vi "SR Scan.vi"() -> ()   [LabVIEW 2012]
uses:
  user.lib/SpectralRadar.llb/Scan Pattern.lvclass
  user.lib/SpectralRadar.llb/Probe.lvclass
  user.lib/SpectralRadar.llb/Coloring.lvclass
  user.lib/SpectralRadar.llb/Colorscheme Selection.ctl
  user.lib/SpectralRadar.llb/ImageField.lvclass
  <vilib>/Utility/error.llb/DialogType.ctl
  user.lib/SpectralRadar.llb/Coloring Byteorder.ctl
  user.lib/SpectralRadar.llb/Probe Parameter Int Selection.ctl
  user.lib/SpectralRadar.llb/Processing Parameter Int Selection.ctl
  user.lib/SpectralRadar.llb/Normal Direction Selection.ctl
  user.lib/SpectralRadar.llb/Colored Data Export Format Selection.ctl
  user.lib/SpectralRadar.llb/Data Export Format Selection.ctl
  user.lib/SpectralRadar.llb/Data Analyzation Selection.ctl
  user.lib/SpectralRadar.llb/display Data 2D.vi
  user.lib/SpectralRadar.llb/display Data 1D in XY-Graph.vi
  user.lib/SpectralRadar.llb/set Scan Output.vi
  user.lib/SpectralRadar.llb/Colored Data.lvclass
  user.lib/SpectralRadar.llb/LabVIEW Helper.lvlib
  user.lib/SpectralRadar.llb/OCT Device.lvclass
  user.lib/SpectralRadar.llb/Processing.lvclass
  user.lib/SpectralRadar.llb/FullRange.lvclass
  user.lib/SpectralRadar.llb/Settings.lvclass
  user.lib/SpectralRadar.llb/FileSelection.lvlib
  user.lib/SpectralRadar.llb/Raw Data.lvclass
  user.lib/SpectralRadar.llb/Data.lvclass
  user.lib/SpectralRadar.llb/Buffer.lvclass
  user.lib/SpectralRadar.llb/Post Processing.lvlib
  user.lib/SpectralRadar.llb/Raw Data Export Format Selection.ctl
panel:
  in  "Average A-scan":bool
  in  "Boolean 2":bool
  in  "Filter Options":bool
  in  "Filter":bool
  in  "B-Scan \nAveraging":i32=1 min=1 max=20 step=1
  in  "BScan angle \n[deg]":dbl(knob) scale=0.0..180.0 scale format="%#.6g"
  in  "BScan\nY offset [mm]":dbl min=-5.0 max=5.0 format="%_4f"
  in  "BScan\nX offset [mm]":dbl min=-5.0 max=5.0 format="%_4f"
  out "ImageField":refnum<class "ImageField.lvclass">
  in  "Auto Range Button":bool
  in  "Image field correction":bool
  out "Save All Progress":i32(slide) min=0 max=35 scale=0.0..11.0
  in  "Palette":T1
  in  "Light":dbl(slide)=51.27999885380268 caption="Sharpness" min=0.0 max=100.0 step=0.009999999776482582 scale=0.0..100.0
  out "Coloring":refnum<class "Coloring.lvclass">
  out "GalvoControl":refnum<class "Probe.lvclass">
  out "Scan Pattern":refnum<class "Scan Pattern.lvclass">
  out "AutoSafe":bool
  in  "Stability":dbl(slide) caption="SNR" min=0.0 max=1.0 step=1.0
  in  "Averaging*Binning":i32(slide)=1 caption="Quality" min=1 max=200 step=1 scale=1.0..200.0
  in  "Options":bool
  in  "Window":T2(ring)
  in  "ShowVideoImage":bool=TRUE caption="Show Video Image"
  out "StreamingPath":path
  in  "Streaming":bool caption="Stream B-Scans"
  out "Image":T3(plugin-control)
  out "Frame Rate":dbl=6.134969234466553 format="%#_3g"
  in  "RunMeasurement":bool
  out "StopIndicator":bool
  in  "Save all":bool
  in  "Brightness":sgl(slide)=0.5272727 caption="Sharpness" min=0 max=1 step=0.01 scale=0.0..1.0
  in  "Contrast":sgl(slide)=0.53333336 caption="Sharpness" min=0 max=1 step=0.01 scale=0.0..1.0
  in  "Saturation":sgl(slide)=0.5212121 caption="Sharpness" min=0 max=1 step=0.01 scale=0.0..1.0
  out "Spacing Z":dbl=2.0 min=1.0 max=500.0 step=1.0 format="%-#2_3f"
  in  "Save":bool
  in  "Description":string
  in  "LowerBScanBorder":dbl=0.972000002861023 min=1.4420210526315789 max=4.806736842105263 step=0.1 format="%.2f"
  in  "UpperBScanBorder":dbl min=0.0 max=0.9613473684210526 step=0.10000000149011612 format="%.2f"
  out "Reference Intensity":sgl(slide) max=140000 scale=0.0..1.0
  out "Next File Name":path=path "D:/OCTData"
  in  "Set Path":bool
  in  "Recallibrate":bool
  in  "Range X [mm]":dbl=2.0 caption="Bereich [mm]" min=0.0 max=10.0 step=0.5 format="%_3f"
  out "Spacing X [µm]":dbl=2.0 min=1.0 max=500.0 step=1.0 format="%#_3g"
  in  "Columns":i32=1000 min=50 max=10240 step=1
  in  "Cursors":bool
  out "Cursor on":bool
  in  "Index of Refraction":dbl=1.0 min=1.0 max=5.0 step=0.10000000149011612 format="%.3f"
  out "Distance Y [mm]":sgl format="%.3f"
  out "Distance X [mm]":sgl format="%.3f"
  out "AScan":cluster{"B-Scan":sgl[], i32[]}(graph)
  in  "Image#":i32=1 caption="of 0" min=1 max=1 step=1
  in  "QuitApp":bool
  in  "Boundries":cluster{sgl, sgl}(slide)={76.65738, 42.00557} scale=15.0..120.0
  out "B-Scan":sgl[][](graph)
  # "Version 5.1"
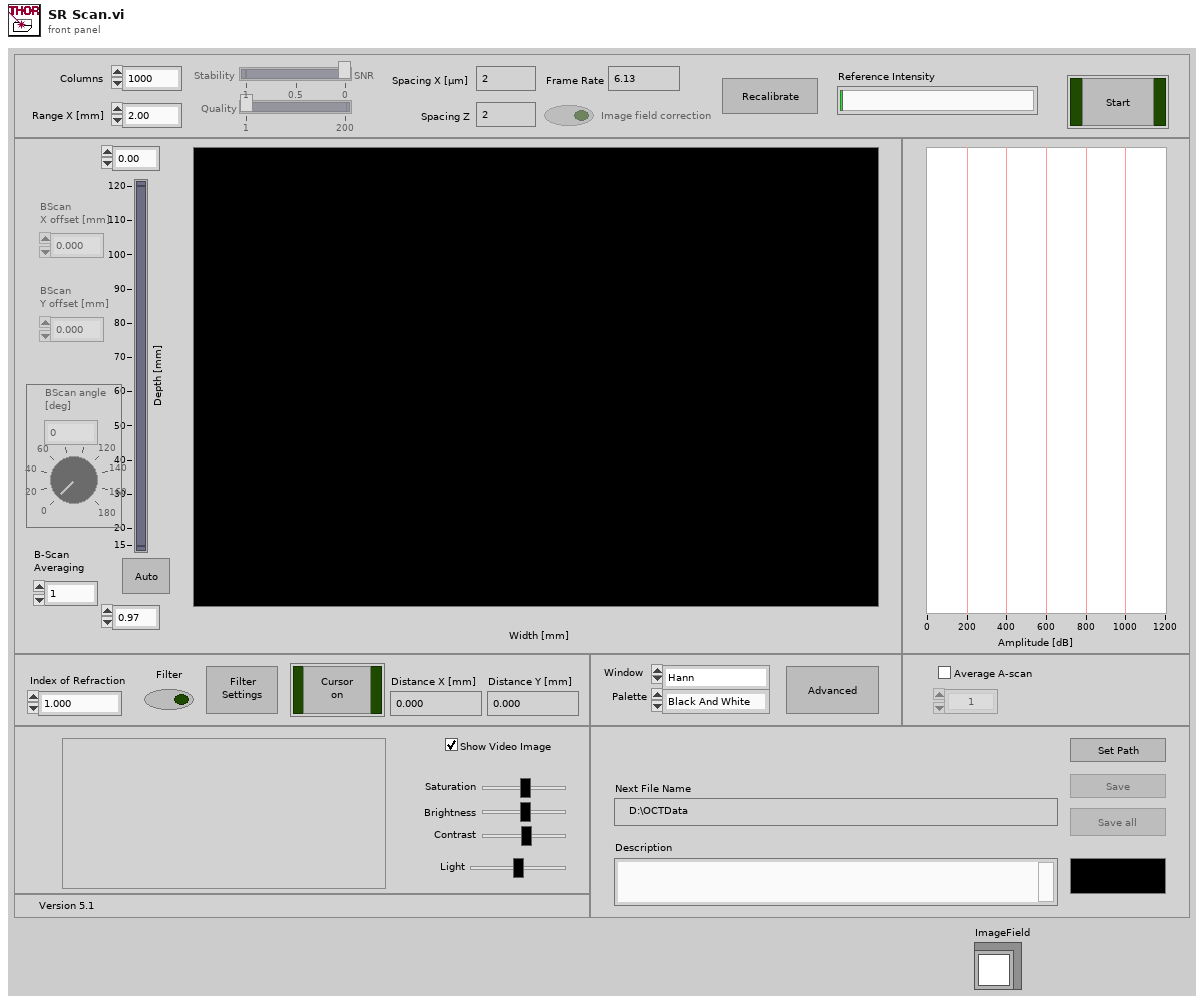
[diagram p1: front panel]
types:
  T1 = typedef "Coloring.lvclass/Colorscheme Selection.ctl" = enum16{"Black And White", "Inverted Black And White", "Color", "Black and Orange", "Black and Red", "Doppler Phase Coloring"}
  T2 = enum16{"Hann", "Hamming", "Gauss", "Tapered Cosine", "Blackman", "4 Term B-Harris"}
  T3 = typedef "IMAQ Image.ctl" = refnum<image>
  T4 = typedef "Coloring.lvclass/Coloring Byteorder.ctl" = enum16{"RGBA32", "BGRA32", "ARGB32", ""}
  T5 = enum16{"Full Well Capacity", "z Spacing", "z Range", "Dynamc Range Min [dB]", "Dynamic Range Low [dB]", "Dynamic Range High [dB]", "Dynamic Range Max [dB]"}
  T6 = typedef "Probe.lvclass/Probe Parameter Int Selection.ctl" = enum16{"Apodization Cycles", "Oversampling", "Oversampling Slow Axis", "Speckle Reduction"}
  T7 = typedef "Processing.lvclass/Processing Parameter Int Selection.ctl" = enum32{"Spectrum Averaging", "A-Scan Averaging", "B-Scan Averaging", "Zero Padding", "Number of Threads", "Fourier Averaging"}
  T8 = typedef "Data.lvclass/Normal Direction Selection.ctl" = enum16{"Direction 1", "Direction 2", "Direction 3"}
  T9 = typedef "Data.lvclass/Data Export Format Selection.ctl" = enum16{"SRM (Spectral Radar Metafile)", "RAW", "CSV", "TXT", "Table TXT", "Fits", "VFF", "VTK", "TIFF"}
  T10 = typedef "Colored Data.lvclass/Colored Data Export Format Selection.ctl" = enum16{"SRM (Spectral Radar Metafile)", "RAW", "BMP", "PNG", "JPG", "PDF", "TIFF"}
  T11 = enum16{"Asynchronous Continuous", "Asynchronous Finite", "Synchronous"}
  T12 = typedef "Data.lvclass/Data Analyzation Selection.ctl" = enum16{"Min", "Mean", "Max"}
  T13 = typedef "Raw Data.lvclass/Raw Data Export Format Selection.ctl" = enum16{"RAW", "SRR (Spectral Radar Raw)"}
  T14 = typedef "DialogType.ctl" = u16
  T15 = typedef "Image Type" = u32
  T16 = enum8{"Enabled", "Disabled", "Disabled and Grayed Out"}
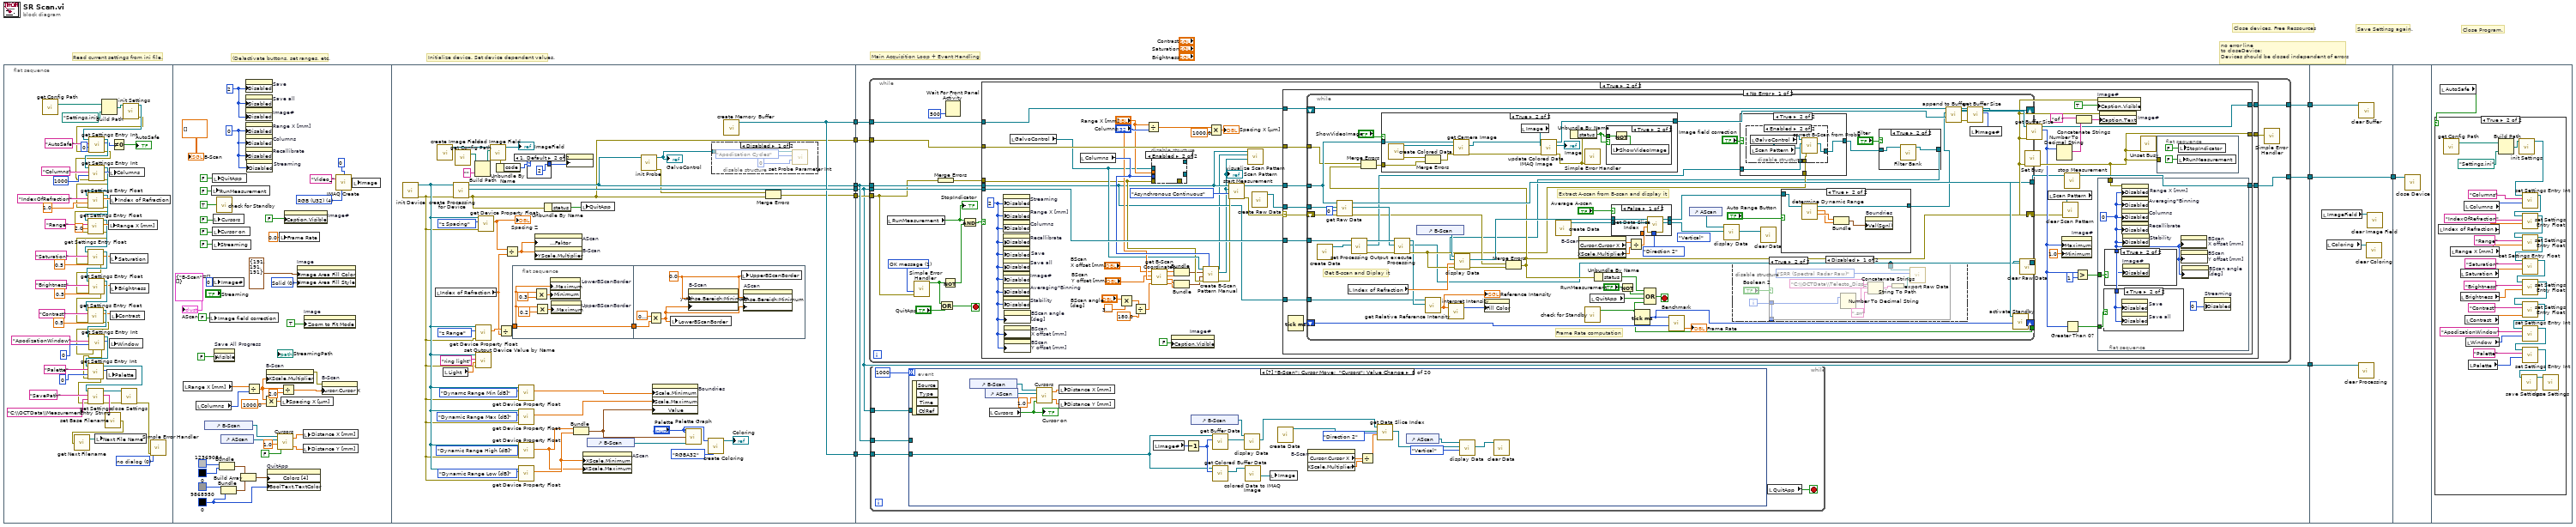
[diagram p0: block diagram]
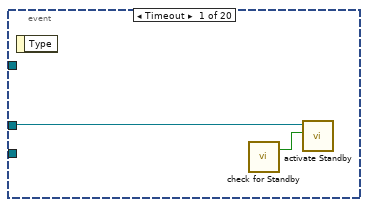
[diagram p4: hidden frame]
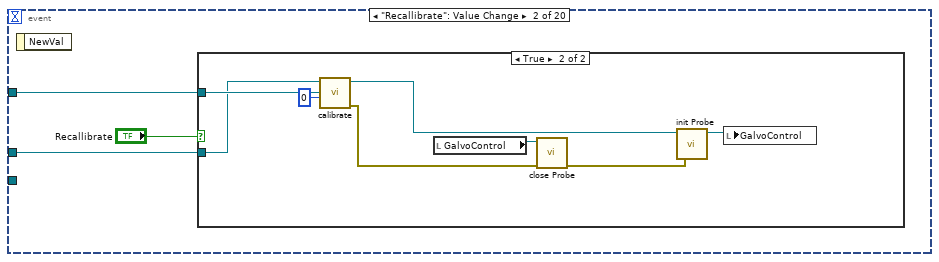
[diagram p5: hidden frame]
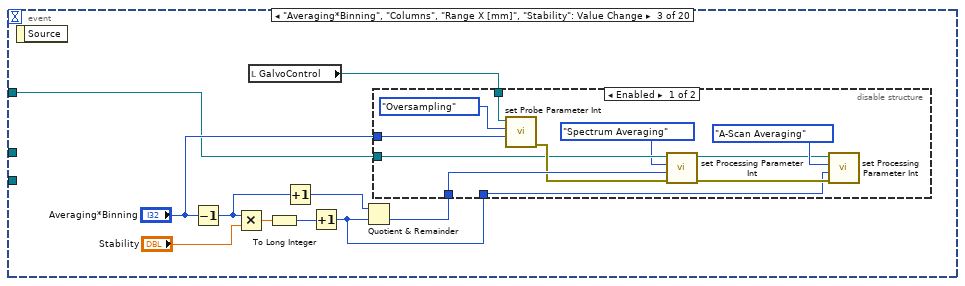
[diagram p7: hidden frame]
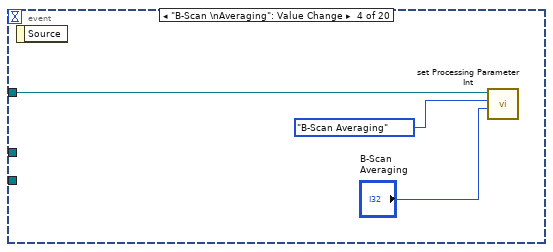
[diagram p9: hidden frame]
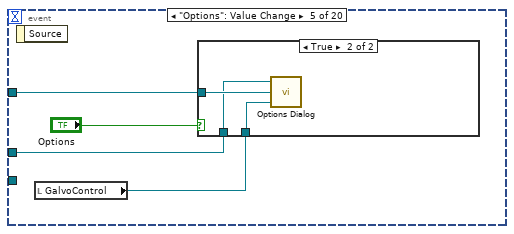
[diagram p10: hidden frame]
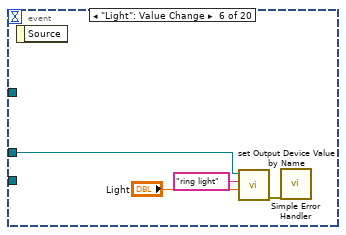
[diagram p12: hidden frame]
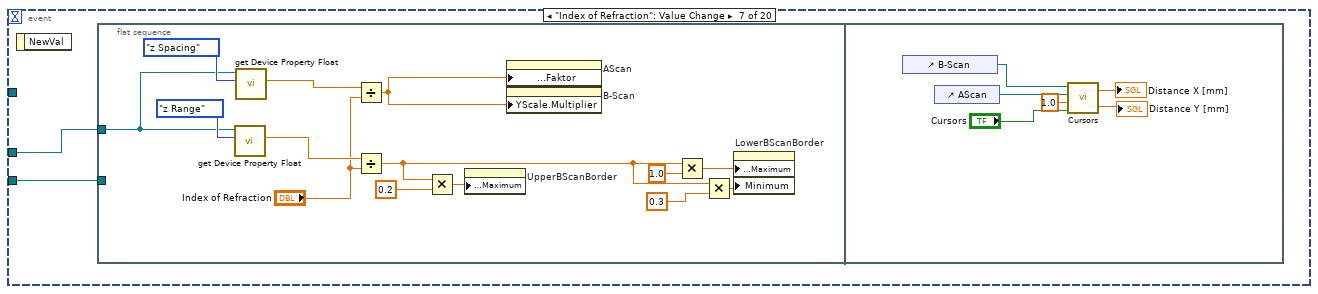
[diagram p13: hidden frame]
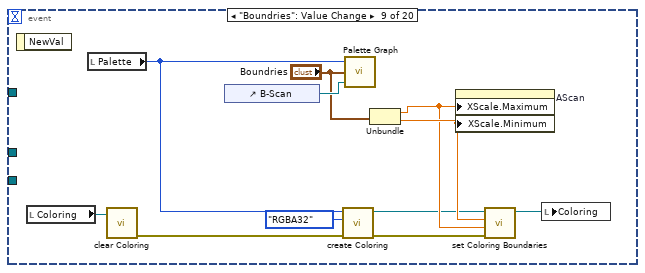
[diagram p14: hidden frame]
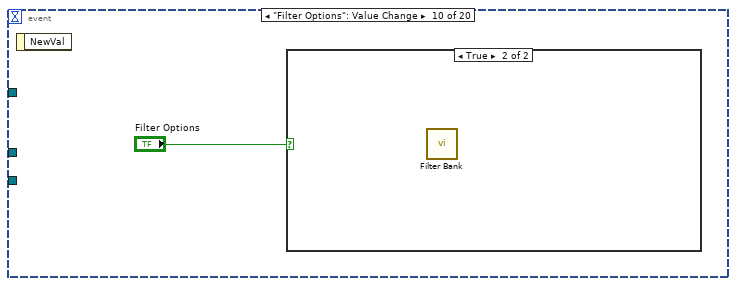
[diagram p15: hidden frame]
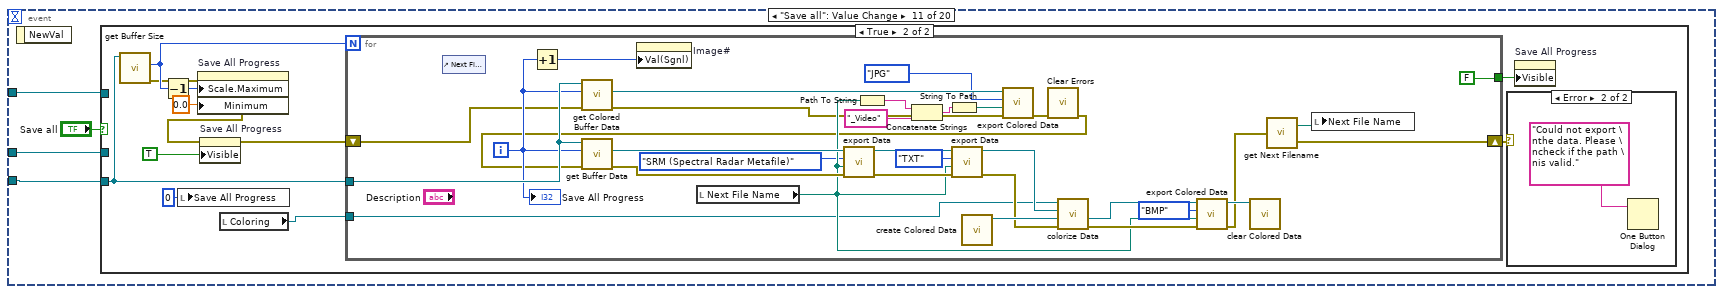
[diagram p17: hidden frame]
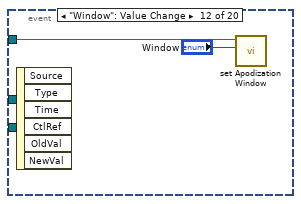
[diagram p20: hidden frame]
diagram:
  # "Close Program."
  # "Save Settinsg again."
  # "Close devices, Free Ressources"
  # "Main Acquisition Loop + Event Handling"
  # "Initialize device. Set device dependent values."
  # "(De)activate buttons, set ranges, etc."
  # "Read current settings from ini file."
  # "no error line\nto closeDevice:\nDevices should be closed independent of errors"
  n1 = flat-sequence {
    tunnel: [w138] -> w10
    tunnel: [w118] -> w7
    tunnel: [w151] -> w6
    tunnel: [w117] -> w4
    tunnel: [w140] -> w3
    tunnel: [w140] -> w1
    tunnel: w10 -> [w175]
    tunnel: [w176] -> w8
    tunnel: w7 -> [w174]
    tunnel: w6 -> [w172]
    tunnel: [w172] -> w5
    tunnel: w4 -> [w173]
    tunnel: w3 -> [w171]
    tunnel: [w170] -> w2
    tunnel: w1 -> [w169]
    tunnel: [w672] -> w9
    tunnel: w8 -> [w672]
    tunnel: w5 -> [w671]
    tunnel: w2 -> [w670]
    tunnel: w9 -> [w673]
    frame #0 {
      w22 = T14 0 items=["no dialog", "OK message", "continue or stop message", "OK message + warnings", "continue/stop + warnings"] ("type of dialog (OK msg:1)")
      n2 = call "get Config Path.vi"() -> ("Path"=w25:path)  [unwired: 1 in, 1 out]
      n3 = Build Path(base path=w25, name or relative path=path "Settings.ini" ("Relative \"SpectralRadar.ini\" Path")) -> (appended path=w69:path)
      n4 = call "init Settings.vi"("Path to settings file"=w69) -> ("error out"=w24:errorcluster, "Settings"=w56:refnum<class "Settings.lvclass">)  [unwired: 5 in]
      n5 = call "get Settings Entry Int.vi"("error in (no error)"=w24, "Default Value"=0, "Node Name"="AutoSafe", "Settings"=w56) -> ("error out"=w19:errorcluster, "Value"=w53:i32, "Settings"=w57:refnum<class "Settings.lvclass">)  [unwired: 1 in]
      n6 = call "get Settings Entry Int.vi"("error in (no error)"=w19, "Default Value"=1000, "Node Name"="Columns", "Settings"=w57) -> ("error out"=w18:errorcluster, "Value"=w67:i32, "Settings"=w59:refnum<class "Settings.lvclass">)  [unwired: 1 in]
      n7 = call "get Settings Entry Float.vi"("error in (no error)"=w18, "Default Value"=1.0, "Node Name"="IndexOfRefraction", "Settings"=w59) -> ("error out"=w17:errorcluster, "Value"=w63:dbl, "Settings"=w58:refnum<class "Settings.lvclass">)  [unwired: 1 in]
      n8 = call "get Settings Entry Float.vi"("error in (no error)"=w17, "Default Value"=2.0, "Node Name"="Range", "Settings"=w58) -> ("error out"=w16:errorcluster, "Value"=w60:dbl, "Settings"=w49:refnum<class "Settings.lvclass">)  [unwired: 1 in]
      n9 = call "get Settings Entry Float.vi"("error in (no error)"=w16, "Default Value"=0.5, "Node Name"="Saturation", "Settings"=w49) -> ("error out"=w15:errorcluster, "Value"=w35:dbl, "Settings"=w46:refnum<class "Settings.lvclass">)  [unwired: 1 in]
      n10 = call "get Settings Entry Float.vi"("error in (no error)"=w15, "Default Value"=0.5, "Node Name"="Brightness", "Settings"=w46) -> ("error out"=w14:errorcluster, "Value"=w34:dbl, "Settings"=w39:refnum<class "Settings.lvclass">)  [unwired: 1 in]
      n11 = call "get Settings Entry Float.vi"("error in (no error)"=w14, "Default Value"=0.5, "Node Name"="Contrast", "Settings"=w39) -> ("error out"=w13:errorcluster, "Value"=w33:dbl, "Settings"=w38:refnum<class "Settings.lvclass">)  [unwired: 1 in]
      n12 = call "get Settings Entry Int.vi"("error in (no error)"=w13, "Default Value"=0, "Node Name"="ApodizationWindow", "Settings"=w38) -> ("error out"=w12:errorcluster, "Value"=w36:i32, "Settings"=w37:refnum<class "Settings.lvclass">)  [unwired: 1 in]
      n13 = call "get Settings Entry Int.vi"("error in (no error)"=w12, "Default Value"=0, "Node Name"="Palette", "Settings"=w37) -> ("error out"=w11:errorcluster, "Value"=w20:i32, "Settings"=w31:refnum<class "Settings.lvclass">)  [unwired: 1 in]
      n14 = call "get Settings Entry String.vi"("error in (no error)"=w11, "Default Value"="C:\\OCTData\\Measurement", "Node Name"="SavePath", "Settings"=w31) -> ("error out"=w23:errorcluster, "Value"=w28:string, "Settings"=w30:refnum<class "Settings.lvclass">)  [unwired: 1 in]
      n15 = call "set Base Filename.vi"("Base"=w28) -> ("error out"=w27:errorcluster)  [unwired: 1 in]
      n16 = call "get Next Filename.vi"("error in (no error)"=w27) -> ("Next File Name"=w26:path)  [unwired: 1 out]
      n17 = local write "Next File Name"(w26) -> ()
      n18 = local write "Palette"(w20) -> ()
      n19 = local write "Range X [mm]"(w60) -> ()
      n20 = local write "Columns"(w67) -> ()
      n21 = local write "Window"(w36) -> ()
      n22 = local write "Index of Refraction"(w63) -> ()
      n23 = local write "Saturation"(w35) -> ()
      n24 = local write "Brightness"(w34) -> ()
      n25 = local write "Contrast"(w33) -> ()
      n26 = Not Equal To 0?(x=w53) -> (x != 0?=→"AutoSafe":bool)
      n27 = call "close Settings.vi"("error in (no error)"=w23, "Settings"=w30) -> ("error out"=w21:errorcluster)  [unwired: 5 in]
      n28 = call <vilib>:"Simple Error Handler.vi"("type of dialog (OK msg:1)"=w22, "error in (no error)"=w21) -> ()  [unwired: 3 in, 5 out]
    }
    frame #1 {
      w77 = T15 4 items=["Grayscale (U8)", "Grayscale (I16)", "Grayscale (SGL)", "Complex (CSG)", "RGB (U32)", "HSL (U32)", "RGB (U64)", "Grayscale (U16)"] ("Image Type")
      w83 = u32 0 items=["Default"=3, "Solid"=0, "Hatch"=2] ("Image Area:Background:Fill Style")
      w104 = u32 0
      w112 = u8 0 ("Deaktiviert")
      w113 = u8 2 ("Deaktiviert")
      n29 = local read "Range X [mm]"() -> (w90:dbl)
      n30 = local read "Columns"() -> (w85:i32)
      n31 = control-ref of="B-Scan"() -> (w93:refnum<vi>)
      n32 = local write "Image field correction"(FALSE ("Confocal correction")) -> ()
      n33 = local write "RunMeasurement"(FALSE ("s/t")) -> ()
      n34 = local write "QuitApp"(FALSE ("QuitApp")) -> ()
      n35 = local write "Cursor on"(FALSE ("Cursor on")) -> ()
      n36 = local write "Streaming"(FALSE ("Streaming")) -> ()
      n37 = local write "Cursors"(FALSE ("Cursors")) -> ()
      n38 = local write "Image#"(0 ("Image#")) -> ()
      n39 = property on="Save All Progress" class="Slide (strict)"("Visible"=FALSE) -> ()  [unwired: 2 in, 2 out]
      n40 = call "check for Standby.vi"("ResetTimer"=TRUE) -> ()  [unwired: 2 out]
      n41 = Bundle(u32 12369084, u32 0) -> (w101:cluster{u32, u32})  [unwired: 1 in]
      n42 = control-ref of="AScan"() -> (w94:refnum<vi>)
      n43 = Bundle(u32 9868950, w104) -> (w102:cluster{u32, u32})  [unwired: 1 in]
      n44 = Build Array(w101, w102) -> (w103:cluster{u32, u32}[])
      n45 = property on="Save" class="Bool"("Disabled"=w113) -> ()  [unwired: 2 in, 2 out]
      n46 = property on="Save all" class="Bool (strict)"("Disabled"=w113) -> ()  [unwired: 2 in, 2 out]
      n47 = property on="Image#" class="DigNum (strict)"("Disabled"=w113) -> ()  [unwired: 2 in, 2 out]
      n48 = property on="Range X [mm]" class="DigNum (strict)"("Disabled"=w112) -> ()  [unwired: 2 in, 2 out]
      n49 = property on="Columns" class="DigNum (strict)"("Disabled"=w112) -> ()  [unwired: 2 in, 2 out]
      n50 = property on="Recallibrate" class="Bool"("Disabled"=w112) -> ()  [unwired: 2 in, 2 out]
      n51 = property on="Streaming" class="Bool (strict)"("Disabled"=w112) -> ()  [unwired: 2 in, 2 out]
      n52 = Divide(x=w90, y=w85) -> (x/y=w88:dbl)
      n53 = Multiply(x=w88, y=1000.0) -> (x*y=w86:dbl)
      n54 = property on="B-Scan" class="IntGraph (strict)"("XScale.Multiplier"=w88) -> (error out=w91:errorcluster)  [unwired: 2 in, 1 out]
      n55 = property on="QuitApp" class="Bool (strict)"("Colors [4]"=w103, "BoolText.TextColor"=w104) -> ()  [unwired: 2 in, 2 out]
      n56 = call "Cursors.vi"("Cursors"=FALSE, "IndexOfRefraction"=sgl 1.0, "ReferenceAScan"=w94, "ReferenceBScan"=w93) -> ("DistanceZ"=w97:sgl, "DistanceX"=w96:sgl)
      n57 = local write "Frame Rate"(0.0 ("Frame Rate")) -> ()
      n58 = Divide(x=w88, y=2.0) -> (x/y=w87:dbl)
      n59 = local write "Spacing X [µm]"(w86) -> ()
      n60 = property on="Image#" class="DigNum (strict)"("Caption.Visible"=FALSE ("Untertitel.Sichtbar")) -> ()  [unwired: 2 in, 2 out]
      n61 = property on="Image" class="ImageControl"("Image Area Fill Color"=cluster{"Red":u8, "Green":u8, "Blue":u8} {"Red"=191, "Green"=191, "Blue"=191} ("Image Area:Background:Fill Color"), "Image Area Fill Style"=w83) -> ()  [unwired: 2 in, 2 out]
      n62 = local write "Distance X [mm]"(w96) -> ()
      n63 = local write "Distance Y [mm]"(w97) -> ()
      n64 = property on="Image" class="ImageControl"("Zoom to Fit Mode"=TRUE) -> ()  [unwired: 2 in, 2 out]
      n65 = property on="B-Scan" class="IntGraph (strict)"(error in=w91, "Cursor.Cursor X"=w87) -> ()  [unwired: 1 in, 2 out]
      n66 = call "IMAQ Create"("Border Size"=0, "Image Name"="Video_", "Image Type"=w77) -> ("New Image"=w79:T3)  [unwired: 2 in, 1 out]
      n67 = local write "Image"(w79) -> ()
      "B-Scan" <- sgl[][] [] ("B-Scan")
      "AScan" <- cluster{"B-Scan":sgl[], i32[]} {"B-Scan"=[], []} ("AScan")
    }
    frame #2 {
      n68 = call "init Device.vi"() -> ("error out"=w114:errorcluster, "OCTDevice"=w124:refnum<class "OCT Device.lvclass">)  [unwired: 6 in]
      n69 = local read "Index of Refraction"() -> (w133:dbl)
      n70 = call "create Image Field.vi"() -> ("ImageField out"=w129:refnum<class "ImageField.lvclass">)  [unwired: 6 in, 1 out]
      n71 = local read "Light"() -> (w130:dbl)
      n72 = call "create Processing for Device.vi"("error in (no error)"=w114, "OCTDevice"=w124) -> ("error out"=w118:errorcluster, "Processing"=w151:refnum<class "Processing.lvclass">, "OCTDevice"=w138:refnum<class "OCT Device.lvclass">)  [unwired: 3 in]
      n73 = call "get Config Path.vi"() -> ("Path"=w128:path)  [unwired: 1 in, 1 out]
      n74 = Build Path(base path=w128, name or relative path="") -> (appended path=w126:path)
      n75 = call "get Device Property Float.vi"("error in (no error)"=w114, "Device Property Float Selection"=T5."z Range", "OCTDevice"=w124) -> ("Value"=w136:dbl)  [unwired: 2 in, 2 out]
      n76 = call "set Output Device Value by Name.vi"("error in (no error)"=w114, "Value"=w130, "Identifier"="ring light", "OCTDevice"=w124) -> ()  [unwired: 2 in, 2 out]
      n77 = call "get Device Property Float.vi"("error in (no error)"=w114, "Device Property Float Selection"=T5."z Spacing", "OCTDevice"=w124) -> ("Value"=w134:dbl)  [unwired: 2 in, 2 out]
      "Spacing Z" <- w134
      n78 = call "load Image Field.vi"("Path"=w126, "ImageField in"=w129) -> ("error out"=w123:errorcluster, "ImageField out"=→"ImageField":refnum<class "ImageField.lvclass">)  [unwired: 4 in]
      n79 = Unbundle By Name(w123) -> ("code"=w122:i32)
      n80 = Divide(x=w136, y=w133) -> (x/y=w132:dbl)
      n81 = Divide(x=w134, y=w133) -> (x/y=w135:dbl)
      n82 = flat-sequence {
        tunnel: w132 -> [w158]
        tunnel: [w158] -> w120
        tunnel: w120 -> [w163]
        frame #0 {
          n83 = Multiply(x=w158, y=0.3) -> (x*y=w162:dbl)
          n84 = Multiply(x=w158, y=0.2) -> (x*y=w160:dbl)
          n85 = property on="LowerBScanBorder" class="DigNum (strict)"("Wertebereich:Maximum"=w158, "Minimum"=w162) -> ()  [unwired: 2 in, 2 out]
          n86 = property on="UpperBScanBorder" class="DigNum (strict)"("Wertebereich:Maximum"=w160) -> ()  [unwired: 2 in, 2 out]
        }
        frame #1 {
          w165 = 0.0 ("y")
          n87 = Multiply(x=0.800000011920929, y=w163) -> (x*y=w166:dbl)
          n88 = local write "LowerBScanBorder"(w166) -> ()
          n89 = property on="B-Scan" class="IntGraph (strict)"("y-Achse.Bereich:Minimum"=w165, "y-Achse.Bereich:Maximum"=w166) -> ()  [unwired: 2 in, 2 out]
          n90 = local write "UpperBScanBorder"(w165) -> ()
          n91 = property on="AScan" class="XYGraph (strict)"("y-Achse.Bereich:Minimum"=w165, "y-Achse.Bereich:Maximum"=w166) -> ()  [unwired: 2 in, 2 out]
        }
      }
      n92 = call "get Device Property Float.vi"("error in (no error)"=w114, "Device Property Float Selection"=T5."Dynamc Range Min [dB]", "OCTDevice"=w124) -> ("Value"=w150:dbl)  [unwired: 2 in, 2 out]
      n93 = call "get Device Property Float.vi"("error in (no error)"=w114, "Device Property Float Selection"=T5."Dynamic Range Max [dB]", "OCTDevice"=w124) -> ("Value"=w149:dbl)  [unwired: 2 in, 2 out]
      n94 = call "get Device Property Float.vi"("error in (no error)"=w114, "Device Property Float Selection"=T5."Dynamic Range High [dB]", "OCTDevice"=w124) -> ("Value"=w141:dbl)  [unwired: 2 in, 2 out]
      n95 = call "get Device Property Float.vi"("error in (no error)"=w114, "Device Property Float Selection"=T5."Dynamic Range Low [dB]", "OCTDevice"=w124) -> ("Value"=w142:dbl)  [unwired: 2 in, 2 out]
      n96 = case shown="1, Default" w122 {
        selector: w122 -> [w167 _]
        tunnel: [w167 2 ("code")] -> w121
        frame 0 {
        }
        frame 1, Default {
        }
      }
      n97 = property on="AScan" class="XYGraph (strict)"("y-Achse.Offset und Faktor:Faktor"=w135) -> ()  [unwired: 2 in, 2 out]
      n98 = property on="B-Scan" class="IntGraph (strict)"("YScale.Multiplier"=w135) -> ()  [unwired: 2 in, 2 out]
      n99 = Unbundle By Name(w118) -> ("status"=w152:bool)
      n100 = property on="Image field correction" class="Bool (strict)"("DisabledEnum"=w121) -> ()  [unwired: 2 in, 2 out]
      n101 = Bundle("Value"=w141, "Value"=w142) -> (w154:cluster{"Value":dbl, "Value":dbl})  [unwired: 1 in]
      n102 = local write "QuitApp"(w152) -> ()
      n103 = property on="AScan" class="XYGraph (strict)"("XScale.Minimum"=w142, "XScale.Maximum"=w141) -> ()  [unwired: 2 in, 2 out]
      n104 = control-ref of="B-Scan"() -> (w153:refnum<vi>)
      n105 = call "init Probe.vi"("OCT Device"=w138) -> ("error out"=w116:errorcluster, "GalvoControl"=w119:refnum<class "Probe.lvclass">)  [unwired: 5 in]
      "GalvoControl" <- w119
      n106 = property on="Boundries" class="Slide (strict)"("Scale.Minimum"=w150, "Scale.Maximum"=w149, "Value"=w154) -> ()  [unwired: 2 in, 2 out]
      n107 = call "Palette Graph.vi"("Reference to the B-scan Graph"=w153, "Boundaries"=w154, "Color Scheme"="Palette") -> ()
      n108 = call "create Coloring.vi"("Color Byte Order"=Coloring_Byteorder."RGBA32", "Color Table Selection"="Palette") -> ("Coloring"=→"Coloring":refnum<class "Coloring.lvclass">)  [unwired: 4 in, 1 out]
      n109 = disable-structure shown="Disabled" {
        disable-tunnel: w119 -> [w157 _]
        frame Disabled {
          n110 = call "set Probe Parameter Int.vi"("Value"=0, "Probe Parameter Int"=Probe_Parameter_Int_Selection."Apodization Cycles", "GalvoControl"=w157) -> ()  [unwired: 3 in, 2 out]
        }
        frame Enabled {
        }
      }
      n111 = call "create Memory Buffer.vi"() -> ("Buffer"=w140:refnum<class "Buffer.lvclass">)  [unwired: 6 in, 1 out]
      n112 = Merge Errors(w116, w118) -> (w117:errorcluster)
    }
    frame #3 {
      n113 = while {
        tunnel: w175 -> [w457]
        tunnel: [w456] -> w176
        tunnel: w174 -> [w455]
        tunnel: w172 -> [w454]
        tunnel: w173 -> [w445]
        tunnel: w171 -> [w449]
        tunnel: [w448] -> w170
        stop <- w459 stop-if-true
        w447 = T14 1 items=["no dialog", "OK message", "continue or stop message", "OK message + warnings", "continue/stop + warnings"] ("type of dialog (OK msg:1)")
        n114 = local read "RunMeasurement"() -> (w452:bool)
        "StopIndicator" <- w452
        n115 = call <vilib>:"Simple Error Handler.vi"("type of dialog (OK msg:1)"=w447, "error in (no error)"=w445) -> ("error?"=w451:bool)  [unwired: 3 in, 4 out]
        n116 = Merge Errors(w445) -> (w446:errorcluster)
        n117 = Or(x=w451, y="QuitApp") -> (x .or. y?=w459:bool)
        n118 = Not(x=w451) -> (.not. x?=w450:bool)
        n119 = Wait For Front Panel Activity(1:500 ("Timeout in ms (-1 kein Timeout)")) -> ()  [unwired: 2 in, 1 out]
        n120 = And(x=w452, y=w450) -> (x .and. y?=w453:bool)
        n121 = case shown="True" w453 {
          tunnel: [w462 w501] -> w461
          tunnel: w457 -> [w464 w467]
          tunnel: [w464 w494] -> w456
          tunnel: w455 -> [_ w493]
          tunnel: w454 -> [_ w492]
          tunnel: w449 -> [w463 w488]
          tunnel: [w463 w487] -> w448
          tunnel: w446 -> [w462 w476]
          frame False {
          }
          frame True {
            w478 = u8 2 ("Deaktiviert")
            n122 = property on="Streaming" class="Bool (strict)"("Disabled"=w478) -> ()  [unwired: 2 in, 2 out]
            n123 = property on="Range X [mm]" class="DigNum (strict)"("Disabled"=w478) -> ()  [unwired: 2 in, 2 out]
            n124 = property on="Columns" class="DigNum (strict)"("Disabled"=w478) -> ()  [unwired: 2 in, 2 out]
            n125 = property on="Recallibrate" class="Bool"("Disabled"=w478) -> ()  [unwired: 2 in, 2 out]
            n126 = property on="Save" class="Bool"("Disabled"=w478) -> ()  [unwired: 2 in, 2 out]
            n127 = property on="Save all" class="Bool (strict)"("Disabled"=w478) -> ()  [unwired: 2 in, 2 out]
            n128 = property on="Image#" class="DigNum (strict)"("Disabled"=w478) -> ()  [unwired: 2 in, 2 out]
            n129 = property on="Averaging*Binning" class="Slide (strict)"("Disabled"=w478) -> ()  [unwired: 2 in, 2 out]
            n130 = property on="Stability" class="Slide (strict)"("Disabled"=w478) -> ()  [unwired: 2 in, 2 out]
            n131 = property on="BScan angle \n[deg]" class="Knob (strict)"("DisabledEnum"=w478) -> ()  [unwired: 2 in, 2 out]
            n132 = property on="BScan\nX offset [mm]" class="DigNum (strict)"("DisabledEnum"=w478) -> ()  [unwired: 2 in, 2 out]
            n133 = property on="BScan\nY offset [mm]" class="DigNum (strict)"("DisabledEnum"=w478) -> ()  [unwired: 2 in, 2 out]
            n134 = local read "GalvoControl"() -> (w477:refnum<class "Probe.lvclass">)
            n135 = local read "Columns"() -> (w486:i32)
            n136 = Multiply(x="BScan angle \n[deg]", y=3.141592653589793) -> (x*y=w481:dbl)
            n137 = Divide(x=w481, y=180.0) -> (x/y=w479:dbl)
            n138 = Divide(x="Range X [mm]", y="Columns") -> (x/y=w498:dbl)
            n139 = disable-structure shown="Enabled" {
              disable-tunnel: "Range X [mm]" -> [w508 _]
              disable-tunnel: [w507 _] -> _
              disable-tunnel: w477 -> [w506 _]
              disable-tunnel: [w505 _] -> _
              disable-tunnel: [w504 _] -> _
              disable-tunnel: w476 -> [w503 _]
              disable-tunnel: w486 -> [w502 _]
              frame Disabled {
                n140 = call "create B-Scan Pattern.vi"("Probe"=w506, "Range"=w508, "AScans"=w502, "error in (no error)"=w503) -> ("Probe"=w504:refnum<class "Probe.lvclass">, "Scan Pattern"=w505:refnum<class "Scan Pattern.lvclass">, "error out"=w507:errorcluster)  [unwired: 1 in]
              }
              frame Enabled {
              }
            }
            n141 = call "get B-Scan Coordinates.vi"("BScan Angle"=w479, "BScan Range"="Range X [mm]", "Offset Y"="BScan\nY offset [mm]", "Offset X"="BScan\nX offset [mm]") -> ("End Y"=w472:dbl, "End X"=w473:dbl, "Start Y"=w474:dbl, "Start X"=w475:dbl)
            n142 = property on="Image#" class="DigNum (strict)"("Caption.Visible"=FALSE ("Untertitel.Sichtbar")) -> ()  [unwired: 2 in, 2 out]
            n143 = Bundle("Start X"=w475, "Start Y"=w474) -> (w471:cluster{"Start X":dbl, "Start Y":dbl})  [unwired: 1 in]
            n144 = Bundle("End X"=w473, "End Y"=w472) -> (w470:cluster{"End X":dbl, "End Y":dbl})  [unwired: 1 in]
            n145 = call "create B-Scan Pattern Manual.vi"("AScans"=w486, "error in (no error)"=w476, "Stop"=w470, "Start"=w471, "Probe in"=w477) -> ("error out"=w484:errorcluster, "Scan Pattern"=w465:refnum<class "Scan Pattern.lvclass">, "Probe out"=w466:refnum<class "Probe.lvclass">)  [unwired: 2 in]
            "Scan Pattern" <- w465
            n146 = Multiply(x=w498, y=1000.0) -> (x*y=→"Spacing X [µm]":dbl)
            n147 = call "start Measurement.vi"("error in (no error)"=w484, "Acquisition Type"=T11."Asynchronous Continuous", "Scan Pattern"=w465, "OCTDevice"=w467) -> ("error out"=w490:errorcluster, "OCTDevice"=w500:refnum<class "OCT Device.lvclass">)  [unwired: 1 in, 1 out]
            n148 = call "visualize Scan Pattern.vi"("Scan Pattern in"=w465, "Probe"=w466, "OCT Device"=w467) -> ()  [unwired: 2 in, 4 out]
            n149 = call "create Raw Data.vi"() -> ("Raw Data"=w491:refnum<class "Raw Data.lvclass">)  [unwired: 6 in, 1 out]
            n150 = case shown="No Error" w490 {
              selector: w490 -> [w520 w662]
              tunnel: [w521 w662] -> w501
              tunnel: w493 -> [w534 _]
              tunnel: w500 -> [w533 w666]
              tunnel: [w525 w665] -> w494
              tunnel: w492 -> [w522 _]
              tunnel: w491 -> [w519 _]
              tunnel: w467 -> [w518 _]
              tunnel: w488 -> [w517 w664]
              tunnel: [w515 w664] -> w487
              frame No Error {
                n151 = Tick Count (ms)() -> (millisecond timer value=w524:u32)
                n152 = while {
                  shift-right: [w600] -> _
                  shift-left: w524 -> [w598]
                  tunnel: w533 -> [w592]
                  tunnel: [w590] -> w523
                  tunnel: [w581] -> w509
                  tunnel: w522 -> [w588]
                  shift-right: [w568] -> w510
                  shift-left: w520 -> [w594]
                  tunnel: w519 -> [w591]
                  tunnel: w518 -> [w554]
                  shift-right: [w578] -> w516
                  shift-left: w517 -> [w580]
                  tunnel: [w548] -> w513
                  tunnel: w534 -> [w569]
                  i -> [w547]
                  stop <- w596 stop-if-true
                  (unwired) enum16{"Horiztonal", "Vertical"}."Vertical" ("Orientation")
                  # "Extract A-scan from B-scan and display it"
                  # "Frame Rate computation"
                  # "Get B-scan and Diplay it"
                  n153 = call "create Data.vi"() -> ("Data"=w587:refnum<class "Data.lvclass">)  [unwired: 6 in, 1 out]
                  n154 = call "get Raw Data.vi"("error in (no error)"=w594, "Camera Index"=0, "RawData in"=w591, "OCTDevice in"=w592) -> ("error out"=w571:errorcluster, "RawData out"=w585:refnum<class "Raw Data.lvclass">, "OCTDevice out"=w581:refnum<class "OCT Device.lvclass">)  [unwired: 1 in]
                  n155 = local read "Index of Refraction"() -> (w574:dbl)
                  n156 = call-poly "set Processing Output.vi"("Data"=w587, "Processing"=w588) -> ("error out"=w583:errorcluster, "Data"=w572:refnum<class "Data.lvclass">, "Processing"=w586:refnum<class "Processing.lvclass">)  [unwired: 3 in]
                  n157 = call "execute Processing.vi"("error in (no error)"=w583, "Raw Data"=w585, "Processing"=w586) -> ("error out"=w556:errorcluster, "Raw Data"=w548:refnum<class "Raw Data.lvclass">, "Processing"=w555:refnum<class "Processing.lvclass">)  [unwired: 2 in]
                  n158 = control-ref of="B-Scan"() -> (w584:refnum<vi>)
                  n159 = call "get Relative Reference Intensity.vi"("Processing"=w555, "OCTDevice"=w554) -> ("Relative Reference Intensity"=w553:dbl)  [unwired: 2 in, 3 out]
                  "Reference Intensity" <- w553
                  n160 = call "interpret Intensity.vi"("Intensity"=w553) -> ("Color"=w552:u32)  [unwired: 1 in, 1 out]
                  n161 = property on="Reference Intensity" class="Slide (strict)"("Fill Color"=w552) -> ()  [unwired: 2 in, 2 out]
                  n162 = call "create Data.vi"() -> ("Data"=w567:refnum<class "Data.lvclass">)  [unwired: 6 in, 1 out]
                  n163 = property on="B-Scan" class="IntGraph (strict)"() -> ("Cursor.Cursor X"=w563:dbl, "XScale.Multiplier"=w562:dbl)  [unwired: 2 in, 2 out]
                  n164 = call "check for Standby.vi"() -> ("TimeOut"=w590:bool)  [unwired: 1 in, 1 out]
                  n165 = local read "QuitApp"() -> (w589:bool)
                  n166 = Not(x="RunMeasurement") -> (.not. x?=w597:bool)
                  n167 = Divide(x=w563, y=w562) -> (x/y=w564:dbl)
                  n168 = Tick Count (ms)() -> (millisecond timer value=w600:u32)
                  n169 = call "Benchmark.vi"("TimeStart"=w598, "TimeFinish"=w600) -> ("AverageFrameRate"=→"Frame Rate":sgl)  [unwired: 2 in, 2 out]
                  n170 = control-ref of="AScan"() -> (w565:refnum<vi>)
                  n171 = disable-structure shown="Disabled" {
                    disable-tunnel: w548 -> [w616 _]
                    disable-tunnel: w547 -> [w614 _]
                    frame Disabled {
                      n172 = case shown="True" "Boolean 2" {
                        tunnel: w616 -> [_ w619]
                        tunnel: w614 -> [_ w617]
                        frame False {
                        }
                        frame True {
                          n173 = Number To Decimal String(number=w617) -> (decimal integer string=w621:string)  [unwired: 1 in]
                          n174 = Concatenate Strings("C:\\OCTData\\Telesto_Disp_" ("string"), w621, ".srr" ("string")) -> (w622:string)
                          n175 = String To Path(string=w622) -> (path=w623:path)
                          n176 = call "export Raw Data.vi"("Export File"=w623, "Raw Data Export Format Selection"=Raw_Data_Export_Format_Selection."SRR (Spectral Radar Raw)", "Data in"=w619) -> ()  [unwired: 3 in, 2 out]
                        }
                      }
                    }
                    frame Enabled {
                    }
                  }
                  n177 = case shown="True" "Image field correction" {
                    tunnel: w572 -> [w634 w637]
                    tunnel: [w634 w636] -> w551
                    tunnel: w556 -> [_ w635]
                    frame False {
                    }
                    frame True {
                      n178 = disable-structure shown="Enabled" {
                        disable-tunnel: w637 -> [w641 w647]
                        disable-tunnel: [w640 w643] -> w636
                        disable-tunnel: w635 -> [w638 w644]
                        frame Disabled {
                          n179 = local read "Scan Pattern"() -> (w642:refnum<class "Scan Pattern.lvclass">)
                          n180 = local read "ImageField"() -> (w639:refnum<class "ImageField.lvclass">)
                          n181 = call "correct Image Field.vi"("error in (no error)"=w638, "ImageField in"=w639, "Data in"=w641, "Scan Pattern in"=w642) -> ("Data out"=w640:refnum<class "Data.lvclass">)  [unwired: 3 out]
                        }
                        frame Enabled {
                          n182 = local read "GalvoControl"() -> (w646:refnum<class "Probe.lvclass">)
                          n183 = local read "Scan Pattern"() -> (w645:refnum<class "Scan Pattern.lvclass">)
                          n184 = call "correct B-Scan from Probe.vi"("error in (no error)"=w644, "Probe in"=w646, "Data in"=w647, "Scan Pattern in"=w645) -> ("Data out"=w643:refnum<class "Data.lvclass">)  [unwired: 3 out]
                        }
                      }
                    }
                  }
                  n185 = case shown="True" "Filter" {
                    tunnel: w551 -> [w625 w627]
                    tunnel: [w625 w626] -> w550
                    frame False {
                    }
                    frame True {
                      n186 = call "Filter Bank.vi"("Data in"=w627) -> ("Data out"=w626:refnum<class "Data.lvclass">)  [unwired: 6 in]
                    }
                  }
                  n187 = call-poly "display Data.vi"("error in (no error)"=w556, "Index of Refraction"=w574, "Data in"=w550, "IntGraph Refnum"=w584) -> ("error out"=w570:errorcluster, "Data out"=w582:refnum<class "Data.lvclass">)  [unwired: 1 in, 1 out]
                  n188 = Merge Errors(w571, w570) -> (w568:errorcluster)
                  n189 = Merge Errors(w569, w568) -> (w575:errorcluster)
                  n190 = case shown="True" "ShowVideoImage" {
                    tunnel: w592 -> [_ w659]
                    tunnel: w575 -> [_ w651]
                    tunnel: [_ w653] -> w557
                    frame False {
                    }
                    frame True {
                      n191 = call "create Colored Data.vi"() -> ("error out"=w652:errorcluster, "Colored Data"=w658:refnum<class "Colored Data.lvclass">)  [unwired: 6 in]
                      n192 = Merge Errors(w652, w651) -> (w650:errorcluster)
                      n193 = call "get Camera Image.vi"("error in (no error)"=w650, "Colored Data in"=w658, "OCTDevice in"=w659) -> ("error out"=w654:errorcluster, "Colored Data out"=w648:refnum<class "Colored Data.lvclass">)  [unwired: 4 in, 1 out]
                      n194 = local read "Image"() -> (w656:T3)
                      n195 = call "update Colored Data IMAQ Image.vi"("error in (no error)"=w654, "Image in"=w656, "Colored Data"=w648) -> ("error out"=w655:errorcluster, "Image out"=→"Image":T3, "Colored Data"=w653:refnum<class "Colored Data.lvclass">)  [unwired: 2 in]
                      n196 = Unbundle By Name(w655) -> ("status"=w649:bool)
                      n197 = call <vilib>:"Simple Error Handler.vi"("error in (no error)"=w655) -> ()  [unwired: 4 in, 5 out]
                      n198 = case shown="True" w649 {
                        tunnel: w649 -> [_ w661]
                        frame False {
                        }
                        frame True {
                          n199 = Not(x=w661) -> (.not. x?=w660:bool)
                          n200 = local write "ShowVideoImage"(w660) -> ()
                        }
                      }
                    }
                  }
                  n201 = Unbundle By Name(w568) -> ("status"=w593:bool)
                  n202 = case shown="False" "Average A-scan" {
                    tunnel: w582 -> [w607 w613]
                    tunnel: w567 -> [w606 w612]
                    tunnel: [w605 w608] -> w566
                    tunnel: w564 -> [w604 _]
                    tunnel: Normal_Direction_Selection."Direction 2" ("Normal Direction") -> [w603 w611]
                    tunnel: [w602 w609] -> w558
                    frame False {
                      n203 = call "get Data Slice Index.vi"("Normal Direction"=w603, "Index"=w604, "Slice"=w606, "Data"=w607) -> ("Slice"=w605:refnum<class "Data.lvclass">, "Data"=w602:refnum<class "Data.lvclass">)  [unwired: 3 in, 1 out]
                    }
                    frame True {
                      n204 = call "get Data Slice Analyzed.vi"("Normal Direction"=w611, "Data Analyzation Selection"=Data_Analyzation_Selection."Mean", "Slice"=w612, "Data"=w613) -> ("Slice"=w608:refnum<class "Data.lvclass">, "Data"=w609:refnum<class "Data.lvclass">)  [unwired: 3 in, 1 out]
                    }
                  }
                  n205 = Compound Arithmetic op=OR(w593, w597, w589, w590) -> (w596:bool)
                  n206 = call-poly "display Data.vi"("Data"=w566, "XYGraph Refnum"=w565) -> ("Data"=w560:refnum<class "Data.lvclass">)  [unwired: 2 in, 3 out]
                  n207 = call "clear Data.vi"("Data"=w560) -> ()  [unwired: 6 in, 1 out]
                  n208 = case shown="True" "Auto Range Button" {
                    tunnel: w558 -> [w628 w633]
                    tunnel: [w628 w632] -> w544
                    frame False {
                    }
                    frame True {
                      n209 = call "determine Dynamic Range.vi"("Data in"=w633) -> ("High"=w631:sgl, "Low"=w630:sgl, "Data out"=w632:refnum<class "Data.lvclass">)  [unwired: 3 in, 1 out]
                      n210 = Bundle("High"=w631, "Low"=w630) -> (w629:cluster{"High":sgl, "Low":sgl})  [unwired: 1 in]
                      n211 = property on="Boundries" class="Slide (strict)"("Val(Sgnl)"=w629) -> ()  [unwired: 2 in, 2 out]
                    }
                  }
                  n212 = call "append to Buffer.vi"("Colored Data"=w557, "Data"=w544, "Buffer in"=w580) -> ("error out"=w577:errorcluster, "Buffer out"=w579:refnum<class "Buffer.lvclass">)  [unwired: 3 in]
                  n213 = call "get Buffer Size.vi"("error in (no error)"=w577, "Buffer in"=w579) -> ("Buffer Size"=w576:i32, "Buffer out"=w578:refnum<class "Buffer.lvclass">)  [unwired: 3 in, 1 out]
                  n214 = local write "Image#"(w576) -> ()
                }
                n215 = call "activate Standby.vi"("StandBy"=w523, "OCTDevice"=w509) -> ()  [unwired: 4 in, 2 out]
                n216 = call "clear Raw Data.vi"("Raw Data"=w513) -> ()  [unwired: 6 in, 1 out]
                n217 = call <vilib>:"Set Busy.vi"("error in (no error)"=w510) -> ("error out"=w521:errorcluster)  [unwired: 9 in, 1 out]
                n218 = call "get Buffer Size.vi"("error in (no error)"=w510, "Buffer in"=w516) -> ("Buffer Size"=w514:i32, "Buffer out"=w515:refnum<class "Buffer.lvclass">)  [unwired: 3 in, 1 out]
                n219 = local read "Scan Pattern"() -> (w511:refnum<class "Scan Pattern.lvclass">)
                n220 = Number To Decimal String(number=w514) -> (decimal integer string=w528:string)  [unwired: 1 in]
                n221 = property on="Image#" class="DigNum (strict)"("Maximum"=w514, "Minimum"=1.0 ("Data Entry Limits:Minimum")) -> ()  [unwired: 2 in, 2 out]
                n222 = call "clear Scan Pattern.vi"("error in (no error)"=w510, "Scan Pattern in"=w511) -> ()  [unwired: 5 in, 1 out]
                n223 = call "stop Measurement.vi"("OCTDevice"=w509) -> ("OCTDevice"=w525:refnum<class "OCT Device.lvclass">)  [unwired: 5 in, 1 out]
                n224 = Greater Than 0?(x=w514) -> (x > 0?=w532:bool)
                n225 = Greater?(x=w514, y=1) -> (0:w530:bool)
                n226 = Concatenate Strings("of " ("String"), w528) -> (w527:string)
                n227 = property on="Image#" class="DigNum (strict)"(error in=w510, "Caption.Visible"=TRUE ("Untertitel.Sichtbar")) -> ()  [unwired: 1 in, 2 out]
                n228 = flat-sequence {
                  tunnel: w532 -> [w539]
                  tunnel: w530 -> [w538]
                  tunnel: w521 -> [w536]
                  frame #0 {
                    w535 = u8 0 ("Deaktiviert")
                    n229 = case shown="True" w539 {
                      tunnel: w535 -> [_ w540]
                      frame False {
                      }
                      frame True {
                        n230 = property on="Save" class="Bool"("Disabled"=w540) -> ()  [unwired: 2 in, 2 out]
                        n231 = property on="Save all" class="Bool (strict)"("Disabled"=w540) -> ()  [unwired: 2 in, 2 out]
                      }
                    }
                    n232 = case shown="True" w538 {
                      tunnel: w535 -> [_ w541]
                      frame False {
                      }
                      frame True {
                        n233 = property on="Image#" class="DigNum (strict)"("Disabled"=w541) -> ()  [unwired: 2 in, 2 out]
                      }
                    }
                    n234 = property on="Range X [mm]" class="DigNum (strict)"(error in=w536, "Disabled"=w535) -> ()  [unwired: 1 in, 2 out]
                    n235 = property on="Averaging*Binning" class="Slide (strict)"("Disabled"=w535) -> ()  [unwired: 2 in, 2 out]
                    n236 = property on="Columns" class="DigNum (strict)"("Disabled"=w535) -> ()  [unwired: 2 in, 2 out]
                    n237 = property on="Recallibrate" class="Bool"("Disabled"=w535) -> ()  [unwired: 2 in, 2 out]
                    n238 = property on="Stability" class="Slide (strict)"("Disabled"=w535) -> ()  [unwired: 2 in, 2 out]
                    n239 = property on="BScan\nX offset [mm]" class="DigNum (strict)"("DisabledEnum"=w535) -> ()  [unwired: 2 in, 2 out]
                    n240 = property on="BScan\nY offset [mm]" class="DigNum (strict)"("DisabledEnum"=w535) -> ()  [unwired: 2 in, 2 out]
                    n241 = property on="BScan angle \n[deg]" class="Knob (strict)"("DisabledEnum"=w535) -> ()  [unwired: 2 in, 2 out]
                    n242 = property on="Streaming" class="Bool (strict)"("Disabled"=u8 0 ("Deaktiviert")) -> ()  [unwired: 2 in, 2 out]
                  }
                }
                n243 = property on="Image#" class="DigNum (strict)"(error in=w510, "Caption.Text"=w527) -> ()  [unwired: 1 in, 2 out]
                n244 = call <vilib>:"Unset Busy.vi"("error in (no error)"=w521) -> ()  [unwired: 10 in, 1 out]
                n245 = flat-sequence {
                  tunnel: w521 -> [_]
                  frame #0 {
                    n246 = local write "RunMeasurement"(FALSE ("StopIndicator")) -> ()
                    n247 = local write "StopIndicator"(FALSE ("StopIndicator")) -> ()
                  }
                }
              }
              frame Error {
                w663 = T16."Enabled" ("Disabled")
                w667 = FALSE ("RunMeasurement")
                n248 = local write "RunMeasurement"(w667) -> ()
                n249 = local write "StopIndicator"(w667) -> ()
                n250 = call "stop Measurement.vi"("OCTDevice"=w666) -> ("OCTDevice"=w665:refnum<class "OCT Device.lvclass">)  [unwired: 5 in, 1 out]
                n251 = property on="Stability" class="Slide (strict)"("DisabledEnum"=w663) -> ()  [unwired: 2 in, 2 out]
                n252 = property on="Averaging*Binning" class="Slide (strict)"("DisabledEnum"=w663) -> ()  [unwired: 2 in, 2 out]
              }
            }
          }
        }
        n253 = call <vilib>:"Simple Error Handler.vi"("error in (no error)"=w461) -> ()  [unwired: 4 in, 5 out]
      }
      n254 = while {
        tunnel: w175 -> [w179]
        tunnel: w172 -> [w178]
        tunnel: w169 -> [w177]
        stop <- w181 stop-if-true
        n255 = event shown="[7] \"B-Scan\": Cursor Move;  \"Cursors\": Value Change" {
          selector: _ -> [_ _ _ _ _ _ _ _ _ _ _ _ _ _ _ _ _ _ _ _]
          dyn-events: _ -> [_ _ _ _ _ _ _ _ _ _ _ _ _ _ _ _ _ _ _ _]
          timeout: 1000 -> [_ _ _ _ _ _ _ _ _ _ _ _ _ _ _ _ _ _ _ _]
          tunnel: w179 -> [w182 w185 _ _ w220 w227 w231 _ _ _ w289 _ _ _ _ _ w378 w396 _ _]
          tunnel: w178 -> [_ w184 w196 w216 w221 _ _ _ _ _ w288 w336 _ _ _ _ _ w395 _ _]
          tunnel: w177 -> [_ _ _ _ _ _ w230 w253 _ _ w287 _ _ _ _ w377 _ w394 _ _]
          event Timeout {
            n256 = event-data() -> ()  [unwired: 1 in, 1 out]
            n257 = call "check for Standby.vi"() -> ("TimeOut"=w183:bool)  [unwired: 1 in, 1 out]
            n258 = call "activate Standby.vi"("StandBy"=w183, "OCTDevice"=w182) -> ()  [unwired: 4 in, 2 out]
          }
          event "Recallibrate": Value Change {
            n259 = event-data() -> ()  [unwired: 1 in, 1 out]
            n260 = case shown="True" "Recallibrate" {
              tunnel: w185 -> [_ w190]
              tunnel: w184 -> [_ w191]
              frame False {
              }
              frame True {
                n261 = call "calibrate.vi"("Camera index"=0, "Processing in"=w191, "OCTDevice"=w190) -> ("error out"=w188:errorcluster, "OCTDevice"=w189:refnum<class "OCT Device.lvclass">)  [unwired: 2 in, 1 out]
                n262 = local read "GalvoControl"() -> (w194:refnum<class "Probe.lvclass">)
                n263 = call "close Probe.vi"("error in (no error)"=w188, "GalvoControl"=w194) -> ("error out"=w193:errorcluster)  [unwired: 5 in]
                n264 = call "init Probe.vi"("error in (no error)"=w193, "OCT Device"=w189) -> ("GalvoControl"=w192:refnum<class "Probe.lvclass">)  [unwired: 4 in, 1 out]
                n265 = local write "GalvoControl"(w192) -> ()
              }
            }
          }
          event "Averaging*Binning", "Columns", "Range X [mm]", "Stability": Value Change {
            n266 = event-data() -> ()  [unwired: 1 in, 1 out]
            n267 = Decrement(x="Averaging*Binning") -> (x-1=w200:i32)
            n268 = Multiply(x=w200, y="Stability") -> (x*y=w203:dbl)
            n269 = local read "GalvoControl"() -> (w195:refnum<class "Probe.lvclass">)
            n270 = To Long Integer(number=w203) -> (32bit integer=w202:i32)
            n271 = Increment(x=w200) -> (x+1=w201:i32)
            n272 = Increment(x=w202) -> (x+1=w198:i32)
            n273 = Quotient & Remainder(x=w201, y=w198) -> (floor(x/y)=w199:i32)  [unwired: 1 out]
            n274 = disable-structure shown="Enabled" {
              disable-tunnel: w195 -> [w215 _]
              disable-tunnel: w199 -> [w213 _]
              disable-tunnel: w198 -> [w210 _]
              disable-tunnel: "Averaging*Binning" -> [w209 _]
              disable-tunnel: w196 -> [w207 _]
              frame Enabled {
                n275 = call "set Probe Parameter Int.vi"("Value"=w209, "Probe Parameter Int"=Probe_Parameter_Int_Selection."Oversampling", "GalvoControl"=w215) -> ("error out"=w208:errorcluster)  [unwired: 3 in, 1 out]
                n276 = call "set Processing Parameter Int.vi"("error in (no error)"=w208, "Value"=w213, "Processing Paramter Int Selection"=Processing_Parameter_Int_Selection."Spectrum Averaging", "Processing in"=w207) -> ("error out"=w211:errorcluster, "Processing out"=w206:refnum<class "Processing.lvclass">)  [unwired: 2 in]
                n277 = call "set Processing Parameter Int.vi"("error in (no error)"=w211, "Value"=w210, "Processing Paramter Int Selection"=Processing_Parameter_Int_Selection."A-Scan Averaging", "Processing in"=w206) -> ()  [unwired: 2 in, 2 out]
              }
              frame Disabled {
              }
            }
          }
          event "B-Scan \nAveraging": Value Change {
            n278 = event-data() -> ()  [unwired: 1 in, 1 out]
            n279 = call "set Processing Parameter Int.vi"("Value"="B-Scan \nAveraging", "Processing Paramter Int Selection"=Processing_Parameter_Int_Selection."B-Scan Averaging", "Processing in"=w216) -> ()  [unwired: 3 in, 2 out]
          }
          event "Options": Value Change {
            n280 = event-data() -> ()  [unwired: 1 in, 1 out]
            n281 = local read "GalvoControl"() -> (w219:refnum<class "Probe.lvclass">)
            n282 = case shown="True" "Options" {
              tunnel: w221 -> [_ w225]
              tunnel: w220 -> [_ w224]
              tunnel: w219 -> [_ w223]
              frame False {
              }
              frame True {
                n283 = call "Options Dialog.vi"("GalvoControl"=w223, "Processing"=w225, "OCT Device"=w224) -> ()  [unwired: 1 in]
              }
            }
          }
          event "Light": Value Change {
            n284 = event-data() -> ()  [unwired: 1 in, 1 out]
            n285 = call "set Output Device Value by Name.vi"("Value"="Light", "Identifier"="ring light", "OCTDevice"=w227) -> ("error out"=w226:errorcluster)  [unwired: 3 in, 1 out]
            n286 = call <vilib>:"Simple Error Handler.vi"("error in (no error)"=w226) -> ()  [unwired: 4 in, 5 out]
          }
          event "Index of Refraction": Value Change {
            n287 = event-data() -> ()  [unwired: 1 in, 1 out]
            n288 = flat-sequence {
              tunnel: w231 -> [w235]
              tunnel: w230 -> [_]
              frame #0 {
                n289 = call "get Device Property Float.vi"("Device Property Float Selection"=T5."z Range", "OCTDevice"=w235) -> ("Value"=w237:dbl)  [unwired: 3 in, 2 out]
                n290 = call "get Device Property Float.vi"("Device Property Float Selection"=T5."z Spacing", "OCTDevice"=w235) -> ("Value"=w233:dbl)  [unwired: 3 in, 2 out]
                n291 = Divide(x=w233, y="Index of Refraction") -> (x/y=w232:dbl)
                n292 = Divide(x=w237, y="Index of Refraction") -> (x/y=w240:dbl)
                n293 = Multiply(x=w240, y=0.2) -> (x*y=w244:dbl)
                n294 = property on="UpperBScanBorder" class="DigNum (strict)"("Wertebereich:Maximum"=w244) -> ()  [unwired: 2 in, 2 out]
                n295 = property on="AScan" class="XYGraph (strict)"("y-Achse.Offset und Faktor:Faktor"=w232) -> ()  [unwired: 2 in, 2 out]
                n296 = property on="B-Scan" class="IntGraph (strict)"("YScale.Multiplier"=w232) -> ()  [unwired: 2 in, 2 out]
                n297 = Multiply(x=w240, y=1.0) -> (x*y=w243:dbl)
                n298 = Multiply(x=w240, y=0.3) -> (x*y=w241:dbl)
                n299 = property on="LowerBScanBorder" class="DigNum (strict)"("Wertebereich:Maximum"=w243, "Minimum"=w241) -> ()  [unwired: 2 in, 2 out]
              }
              frame #1 {
                n300 = control-ref of="B-Scan"() -> (w250:refnum<vi>)
                n301 = control-ref of="AScan"() -> (w249:refnum<vi>)
                n302 = call "Cursors.vi"("Cursors"="Cursors", "IndexOfRefraction"=sgl 1.0, "ReferenceAScan"=w249, "ReferenceBScan"=w250) -> ("DistanceZ"=→"Distance Y [mm]":sgl, "DistanceX"=→"Distance X [mm]":sgl)
              }
            }
          }
          event "B-Scan": Cursor Move; "Cursors": Value Change {
            n303 = event-data() -> ()  [unwired: 1 in, 4 out]
            n304 = control-ref of="B-Scan"() -> (w273:refnum<vi>)
            n305 = control-ref of="AScan"() -> (w272:refnum<vi>)
            n306 = local read "Cursors"() -> (w269:bool)
            "Cursor on" <- w269
            n307 = call "Cursors.vi"("Cursors"=w269, "IndexOfRefraction"=sgl 1.0, "ReferenceAScan"=w272, "ReferenceBScan"=w273) -> ("DistanceZ"=w270:sgl, "DistanceX"=w271:sgl)
            n308 = local write "Distance X [mm]"(w271) -> ()
            n309 = local write "Distance Y [mm]"(w270) -> ()
            n310 = local read "Image#"() -> (w254:i32)
            n311 = Decrement(x=w254) -> (x-1=w255:i32)
            n312 = control-ref of="B-Scan"() -> (w267:refnum<vi>)
            n313 = call "get Buffer Data.vi"("Index"=w255, "Buffer in"=w253) -> ("Data out"=w268:refnum<class "Data.lvclass">)  [unwired: 3 in, 2 out]
            n314 = call "get Colored Buffer Data.vi"("Index"=w255, "Buffer in"=w253) -> ("Colored Data"=w266:refnum<class "Colored Data.lvclass">)  [unwired: 3 in, 2 out]
            n315 = call-poly "display Data.vi"("Data in"=w268, "IntGraph Refnum"=w267) -> ("Data out"=w262:refnum<class "Data.lvclass">)  [unwired: 3 in, 2 out]
            n316 = call "colored Data to IMAQ Image.vi"("Colored Data"=w266) -> ("Image Out"=w265:T3)  [unwired: 4 in, 2 out]
            n317 = local write "Image"(w265) -> ()
            n318 = call "create Data.vi"() -> ("Data"=w263:refnum<class "Data.lvclass">)  [unwired: 6 in, 1 out]
            n319 = property on="B-Scan" class="IntGraph (strict)"() -> ("Cursor.Cursor X"=w258:dbl, "XScale.Multiplier"=w257:dbl)  [unwired: 2 in, 2 out]
            n320 = Divide(x=w258, y=w257) -> (x/y=w256:dbl)
            n321 = call "get Data Slice Index.vi"("Normal Direction"=Normal_Direction_Selection."Direction 2", "Index"=w256, "Slice"=w263, "Data"=w262) -> ("Slice"=w261:refnum<class "Data.lvclass">)  [unwired: 3 in, 2 out]
            n322 = control-ref of="AScan"() -> (w260:refnum<vi>)
            n323 = call-poly "display Data.vi"("Orientation"=enum16{"Horizontal", "Vertical"}."Vertical", "Data"=w261, "XYGraph Refnum"=w260) -> ("Data"=w259:refnum<class "Data.lvclass">)  [unwired: 1 in, 3 out]
            n324 = call "clear Data.vi"("Data"=w259) -> ()  [unwired: 6 in, 1 out]
          }
          event "Boundries": Value Change {
            n325 = event-data() -> ()  [unwired: 1 in, 1 out]
            n326 = local read "Coloring"() -> (w279:refnum<class "Coloring.lvclass">)
            n327 = local read "Palette"() -> (w281:T1)
            n328 = call "clear Coloring.vi"("Coloring"=w279) -> ("error out"=w276:errorcluster)  [unwired: 6 in]
            n329 = control-ref of="B-Scan"() -> (w285:refnum<vi>)
            n330 = call "create Coloring.vi"("error in (no error)"=w276, "Color Byte Order"=Coloring_Byteorder."RGBA32", "Color Table Selection"=w281) -> ("error out"=w277:errorcluster, "Coloring"=w280:refnum<class "Coloring.lvclass">)  [unwired: 3 in]
            n331 = call "Palette Graph.vi"("Reference to the B-scan Graph"=w285, "Boundaries"="Boundries", "Color Scheme"=w281) -> ()
            n332 = Unbundle("Boundries") -> (w282:sgl, w283:sgl)
            n333 = property on="AScan" class="XYGraph (strict)"("XScale.Maximum"=w282, "XScale.Minimum"=w283) -> ()  [unwired: 2 in, 2 out]
            n334 = call "set Coloring Boundaries.vi"("error in (no error)"=w277, "Danymic Range High [dB]"=w282, "Dynamic Range Low [dB]"=w283, "Coloring in"=w280) -> ("Coloring out"=w278:refnum<class "Coloring.lvclass">)  [unwired: 2 in, 1 out]
            n335 = local write "Coloring"(w278) -> ()
          }
          event "Filter Options": Value Change {
            n336 = event-data() -> ()  [unwired: 1 in, 1 out]
            n337 = case shown="True" "Filter Options" {
              frame False {
              }
              frame True {
                n338 = call "Filter Bank.vi"() -> ()  [unwired: 7 in, 1 out]
              }
            }
          }
          event "Save all": Value Change {
            n339 = event-data() -> ()  [unwired: 1 in, 1 out]
            n340 = case shown="True" "Save all" {
              tunnel: w289 -> [_ _]
              tunnel: w288 -> [_ _]
              tunnel: w287 -> [_ w302]
              frame False {
              }
              frame True {
                n341 = call "get Buffer Size.vi"("Buffer in"=w302) -> ("error out"=w296:errorcluster, "Buffer Size"=w301:i32)  [unwired: 4 in, 1 out]
                n342 = Decrement(x=w301) -> (x-1=w295:i32)
                n343 = local write "Save All Progress"(0 ("Save All Progress")) -> ()
                n344 = property on="Save All Progress" class="Slide (strict)"(error in=w296, "Scale.Maximum"=w295, "Minimum"=0.0 ("Data Entry Limits:Minimum")) -> (error out=w297:errorcluster)  [unwired: 1 in, 1 out]
                n345 = property on="Save All Progress" class="Slide (strict)"(error in=w297, "Visible"=TRUE) -> (error out=w293:errorcluster)  [unwired: 1 in, 1 out]
                n346 = local read "Coloring"() -> (w291:refnum<class "Coloring.lvclass">)
                n347 = for {
                  N: w301 -> [_]
                  tunnel: w302 -> [w316]
                  tunnel: w291 -> [w315]
                  tunnel: [FALSE ("Visible")] -> w298
                  shift-right: [w309] -> w292
                  shift-left: w293 -> [w307]
                  i -> [w312]
                  n348 = control-ref of="Next File Name"() -> ()  [unwired: 1 out]
                  n349 = Increment(x=w312) -> (x+1=w314:i32)
                  n350 = call "get Colored Buffer Data.vi"("error in (no error)"=w307, "Index"=w312, "Buffer in"=w316) -> ("error out"=w313:errorcluster, "Colored Data"=w323:refnum<class "Colored Data.lvclass">)  [unwired: 2 in, 1 out]
                  n351 = property on="Image#" class="DigNum (strict)"("Val(Sgnl)"=w314) -> ()  [unwired: 2 in, 2 out]
                  n352 = local read "Next File Name"() -> (w321:path)
                  n353 = Path To String(path=w321) -> (string=w320:string)
                  n354 = Concatenate Strings(w320, "_Video" ("name or relative path")) -> (w318:string)
                  n355 = String To Path(string=w318) -> (path=w317:path)
                  n356 = call "create Colored Data.vi"() -> ("Colored Data"=w329:refnum<class "Colored Data.lvclass">)  [unwired: 6 in, 1 out]
                  n357 = call "export Colored Data.vi"("error in (no error)"=w313, "File Name"=w317, "Colored Data Export Format Selection"=Colored_Data_Export_Format_Selection."JPG", "Colored Data in"=w323) -> ("error out"=w308:errorcluster)  [unwired: 2 in, 1 out]
                  n358 = call <vilib>:"Clear Errors.vi"("error in (no error)"=w308) -> ("error out"=w306:errorcluster)  [unwired: 6 in]
                  n359 = call "get Buffer Data.vi"("error in (no error)"=w306, "Index"=w312, "Buffer in"=w316) -> ("error out"=w333:errorcluster, "Data out"=w334:refnum<class "Data.lvclass">)  [unwired: 2 in, 1 out]
                  n360 = call "export Data.vi"("error in (no error)"=w333, "Export File"=w321, "Data Export Format Selection"=Data_Export_Format_Selection."SRM (Spectral Radar Metafile)", "Data in"=w334) -> ("error out"=w331:errorcluster, "Data out"=w332:refnum<class "Data.lvclass">)  [unwired: 2 in]
                  n361 = call "export Data.vi"("error in (no error)"=w331, "Export File"=w321, "Data Export Format Selection"=Data_Export_Format_Selection."TXT", "Data in"=w332) -> ("error out"=w328:errorcluster, "Data out"=w330:refnum<class "Data.lvclass">)  [unwired: 2 in]
                  n362 = call "colorize Data.vi"("error in (no error)"=w328, "Colored Data"=w329, "Data"=w330, "Coloring in"=w315) -> ("error out"=w325:errorcluster, "Colored Data"=w327:refnum<class "Colored Data.lvclass">)  [unwired: 2 out]
                  n363 = call "export Colored Data.vi"("error in (no error)"=w325, "File Name"=w321, "Colored Data Export Format Selection"=Colored_Data_Export_Format_Selection."BMP", "Colored Data in"=w327) -> ("error out"=w310:errorcluster, "Colored Data out"=w324:refnum<class "Colored Data.lvclass">)  [unwired: 2 in]
                  n364 = call "clear Colored Data.vi"("Colored Data"=w324) -> ()  [unwired: 6 in, 1 out]
                  n365 = call "get Next Filename.vi"("error in (no error)"=w310) -> ("Next File Name"=w335:path, "error out"=w309:errorcluster)
                  n366 = local write "Next File Name"(w335) -> ()
                  "Save All Progress" <- w312
                }
                n367 = case shown="Error" w292 {
                  frame No Error {
                  }
                  frame Error {
                    n368 = One Button Dialog(message="Could not export \nthe data. Please \ncheck if the path \nis valid.") -> ()  [unwired: 1 in, 1 out]
                  }
                }
                n369 = property on="Save All Progress" class="Slide (strict)"("Visible"=w298) -> ()  [unwired: 2 in, 2 out]
              }
            }
          }
          event "Window": Value Change {
            n370 = event-data() -> ()  [unwired: 1 in, 6 out]
            n371 = call "set Apodization Window.vi"("Window"="Window", "Processing"=w336) -> ()  [unwired: 4 in, 2 out]
          }
          event "UpperBScanBorder", "LowerBScanBorder": Value Change {
            n372 = event-data() -> ()  [unwired: 1 in, 1 out]
            n373 = property on="B-Scan" class="IntGraph (strict)"("YScale.Minimum"="UpperBScanBorder", "YScale.Maximum"="LowerBScanBorder") -> ()  [unwired: 2 in, 2 out]
            n374 = property on="AScan" class="XYGraph (strict)"("YScale.Minimum"="UpperBScanBorder", "YScale.Maximum"="LowerBScanBorder") -> ()  [unwired: 2 in, 2 out]
          }
          event "QuitApp": Mouse Enter {
            n375 = event-data() -> ("Time"=w343:u32)  [unwired: 1 in]
            n376 = Tick Count (ms)() -> (millisecond timer value=w344:u32)
            n377 = Subtract(x=w344, y=w343) -> (x-y=w342:u32)
            n378 = Less?(x=w342, y=u32 200) -> (x < y?=w340:bool)
            n379 = case shown="True" w340 {
              frame False {
              }
              frame True {
                w345 = u32 16448250
                n380 = Bundle(u32 16711680, u32 16448250) -> (w347:cluster{u32, u32})  [unwired: 1 in]
                n381 = Bundle(u32 8978432, w345) -> (w346:cluster{u32, u32})  [unwired: 1 in]
                n382 = Build Array(w347, w346) -> (w349:cluster{u32, u32}[])
                n383 = property on="QuitApp" class="Bool (strict)"("Colors [4]"=w349, "BoolText.TextColor"=w345) -> ()  [unwired: 2 in, 2 out]
              }
            }
          }
          event "QuitApp": Mouse Leave {
            w352 = u32 0
            n384 = event-data() -> ()  [unwired: 1 in, 1 out]
            n385 = Bundle(u32 9868950, w352) -> (w353:cluster{u32, u32})  [unwired: 1 in]
            n386 = Bundle(u32 12369084, u32 0) -> (w354:cluster{u32, u32})  [unwired: 1 in]
            n387 = Build Array(w354, w353) -> (w358:cluster{u32, u32}[])
            n388 = property on="QuitApp" class="Bool (strict)"("Colors [4]"=w358, "BoolText.TextColor"=w352) -> ()  [unwired: 2 in, 2 out]
          }
          event "Image#": Value Change {
            n389 = event-data() -> ()  [unwired: 1 in, 1 out]
            n390 = Decrement(x="Image#") -> (x-1=w364:i32)
            n391 = call "get Buffer Data.vi"("Index"=w364, "Buffer in"=w377) -> ("Data out"=w375:refnum<class "Data.lvclass">)  [unwired: 3 in, 2 out]
            n392 = call "get Colored Buffer Data.vi"("Index"=w364, "Buffer in"=w377) -> ("Colored Data"=w363:refnum<class "Colored Data.lvclass">)  [unwired: 3 in, 2 out]
            n393 = local read "Index of Refraction"() -> (w360:dbl)
            n394 = control-ref of="B-Scan"() -> (w374:refnum<vi>)
            n395 = local read "Image"() -> (w361:T3)
            n396 = call "update Colored Data IMAQ Image.vi"("Image in"=w361, "Colored Data"=w363) -> ("Image out"=w362:T3)  [unwired: 3 in, 2 out]
            n397 = call-poly "display Data.vi"("Index of Refraction"=w360, "Data in"=w375, "IntGraph Refnum"=w374) -> ("Data out"=w371:refnum<class "Data.lvclass">)  [unwired: 2 in, 2 out]
            n398 = local write "Image"(w362) -> ()
            n399 = call "create Data.vi"() -> ("Data"=w372:refnum<class "Data.lvclass">)  [unwired: 6 in, 1 out]
            n400 = property on="B-Scan" class="IntGraph (strict)"() -> ("Cursor.Cursor X"=w367:dbl, "XScale.Multiplier"=w366:dbl)  [unwired: 2 in, 2 out]
            n401 = Divide(x=w367, y=w366) -> (x/y=w365:dbl)
            n402 = call "get Data Slice Index.vi"("Normal Direction"=Normal_Direction_Selection."Direction 2", "Index"=w365, "Slice"=w372, "Data"=w371) -> ("Slice"=w370:refnum<class "Data.lvclass">)  [unwired: 3 in, 2 out]
            n403 = control-ref of="AScan"() -> (w369:refnum<vi>)
            n404 = call-poly "display Data.vi"("Orientation"=enum16{"Horizontal", "Vertical"}."Horizontal", "Data"=w370, "XYGraph Refnum"=w369) -> ("Data"=w368:refnum<class "Data.lvclass">)  [unwired: 1 in, 3 out]
            n405 = call "clear Data.vi"("Data"=w368) -> ()  [unwired: 6 in, 1 out]
          }
          event "Set Path": Value Change {
            n406 = event-data() -> ()  [unwired: 1 in, 1 out]
            n407 = case shown="True" "Set Path" {
              tunnel: w378 -> [_ _]
              frame False {
              }
              frame True {
                n408 = local read "Next File Name"() -> (w382:path)
                n409 = File Dialog(4:"SpectralRadar Measurement File" ("pattern label"), 5:"Select" ("button label"), 6:"*.srm" ("pattern"), 7:"Select SpectralRadar Measurement" ("Abfrage"), 9:"Measurement" ("Standardname"), 11:w382) -> (1:w380:bool, 3:w381:path)  [unwired: 1 in, 2 out]
                n410 = case shown="False" w380 {
                  tunnel: w381 -> [w390 _]
                  frame False {
                    n411 = Path To String(path=w390) -> (string=w389:string)
                    n412 = call "set Base Filename.vi"("Base"=w389) -> ("error out"=w391:errorcluster)  [unwired: 1 in]
                    n413 = call "get Next Filename.vi"("error in (no error)"=w391) -> ("Next File Name"=→"Next File Name":path)  [unwired: 1 out]
                  }
                  frame True {
                  }
                }
              }
            }
          }
          event "Save": Value Change {
            n414 = event-data() -> ()  [unwired: 1 in, 1 out]
            n415 = local read "Coloring"() -> (w392:refnum<class "Coloring.lvclass">)
            n416 = case shown="True" "Save" {
              tunnel: w396 -> [_ _]
              tunnel: w395 -> [_ _]
              tunnel: w394 -> [_ w424]
              tunnel: w392 -> [_ w420]
              tunnel: [_ w401] -> w393
              frame False {
              }
              frame True {
                # "No camera image available is not severe. Suppress."
                n417 = local read "Image#"() -> (w425:i32)
                n418 = Decrement(x=w425) -> (x-1=w430:i32)
                n419 = Increment(x=w425) -> (x+1=w422:i32)
                n420 = call "get Buffer Size.vi"("Buffer in"=w424) -> ("Buffer Size"=w423:i32)  [unwired: 4 in, 2 out]
                n421 = call "get Colored Buffer Data.vi"("Index"=w430, "Buffer in"=w424) -> ("error out"=w405:errorcluster, "Colored Data"=w412:refnum<class "Colored Data.lvclass">)  [unwired: 3 in, 1 out]
                n422 = Max & Min(x=w422, y=w423) -> (min(x,y)=w421:i32)  [unwired: 1 out]
                n423 = local read "Next File Name"() -> (w410:path)
                n424 = property on="Image#" class="DigNum (strict)"("Val(Sgnl)"=w421) -> ()  [unwired: 2 in, 2 out]
                n425 = Path To String(path=w410) -> (string=w409:string)
                n426 = Concatenate Strings(w409, "_Video" ("name or relative path")) -> (w407:string)
                n427 = String To Path(string=w407) -> (path=w406:path)
                n428 = call "create Colored Data.vi"() -> ("Colored Data"=w418:refnum<class "Colored Data.lvclass">)  [unwired: 6 in, 1 out]
                n429 = call "export Colored Data.vi"("error in (no error)"=w405, "File Name"=w406, "Colored Data Export Format Selection"=Colored_Data_Export_Format_Selection."JPG", "Colored Data in"=w412) -> ("error out"=w403:errorcluster)  [unwired: 2 in, 1 out]
                n430 = call <vilib>:"Clear Errors.vi"("error in (no error)"=w403) -> ("error out"=w402:errorcluster)  [unwired: 6 in]
                n431 = call "get Buffer Data.vi"("error in (no error)"=w402, "Index"=w430, "Buffer in"=w424) -> ("error out"=w428:errorcluster, "Data out"=w429:refnum<class "Data.lvclass">)  [unwired: 2 in, 1 out]
                n432 = call "export Data.vi"("error in (no error)"=w428, "Export File"=w410, "Data Export Format Selection"=Data_Export_Format_Selection."SRM (Spectral Radar Metafile)", "Data in"=w429) -> ("error out"=w426:errorcluster, "Data out"=w427:refnum<class "Data.lvclass">)  [unwired: 2 in]
                n433 = call "export Data.vi"("error in (no error)"=w426, "Export File"=w410, "Data Export Format Selection"=Data_Export_Format_Selection."TXT", "Data in"=w427) -> ("error out"=w417:errorcluster, "Data out"=w419:refnum<class "Data.lvclass">)  [unwired: 2 in]
                n434 = call "colorize Data.vi"("error in (no error)"=w417, "Colored Data"=w418, "Data"=w419, "Coloring in"=w420) -> ("error out"=w414:errorcluster, "Colored Data"=w416:refnum<class "Colored Data.lvclass">)  [unwired: 2 out]
                n435 = call "export Colored Data.vi"("error in (no error)"=w414, "File Name"=w410, "Colored Data Export Format Selection"=Colored_Data_Export_Format_Selection."BMP", "Colored Data in"=w416) -> ("error out"=w404:errorcluster, "Colored Data out"=w413:refnum<class "Colored Data.lvclass">)  [unwired: 2 in]
                n436 = call "clear Colored Data.vi"("Colored Data"=w413) -> ()  [unwired: 6 in, 1 out]
                n437 = call "get Next Filename.vi"("error in (no error)"=w404) -> ("Next File Name"=w431:path, "error out"=w401:errorcluster)
                n438 = local write "Next File Name"(w431) -> ()
              }
            }
            n439 = case shown="Error" w393 {
              frame No Error {
              }
              frame Error {
                n440 = One Button Dialog(message="Could not export \nthe data. Please \ncheck if the path \nis valid.") -> ()  [unwired: 1 in, 1 out]
              }
            }
          }
          event Mouse Down; Mouse Up {
            n441 = event-data() -> ()  [unwired: 1 in, 1 out]
            n442 = call "check for Standby.vi"("ResetTimer"=TRUE) -> ()  [unwired: 2 out]
          }
          event "AScan": Cursor Move {
            n443 = event-data() -> ()  [unwired: 1 in, 1 out]
            n444 = property on="AScan" class="XYGraph (strict)"("Active Cursor"=u32 0 ("Aktiver Cursor"), "Active Cursor"=u32 1 ("Aktiver Cursor")) -> ("Cursor.Cursor Y"=w442:dbl, "Cursor.Cursor Y"=w441:dbl)  [unwired: 2 in, 2 out]
            n445 = property on="B-Scan" class="IntGraph (strict)"("Active Cursor"=u32 0 ("Aktiver Cursor"), "Cursor.Cursor Y"=w442, "Active Cursor"=u32 1 ("Aktiver Cursor"), "Cursor.Cursor Y"=w441) -> ()  [unwired: 2 in, 2 out]
            n446 = local read "Index of Refraction"() -> (w438:dbl)
            n447 = control-ref of="B-Scan"() -> (w433:refnum<vi>)
            n448 = control-ref of="AScan"() -> (w437:refnum<vi>)
            n449 = local read "Cursors"() -> (w436:bool)
            n450 = call "Cursors.vi"("Cursors"=w436, "IndexOfRefraction"=w438, "ReferenceAScan"=w437, "ReferenceBScan"=w433) -> ("DistanceZ"=w434:sgl, "DistanceX"=w435:sgl)
            n451 = local write "Distance X [mm]"(w435) -> ()
            n452 = local write "Distance Y [mm]"(w434) -> ()
            n453 = local write "Cursor on"(w436) -> ()
          }
        }
        n454 = local read "QuitApp"() -> (w181:bool)
      }
    }
    frame #4 {
      n455 = local read "ImageField"() -> (w668:refnum<class "ImageField.lvclass">)
      n456 = local read "Coloring"() -> (w669:refnum<class "Coloring.lvclass">)
      n457 = call "clear Processing.vi"("Processing"=w671) -> ()  [unwired: 6 in, 1 out]
      n458 = call "clear Buffer.vi"("Buffer"=w670) -> ()  [unwired: 6 in, 1 out]
      n459 = call "clear Coloring.vi"("Coloring"=w669) -> ()  [unwired: 6 in, 1 out]
      n460 = call "clear Image Field.vi"("ImageField in"=w668) -> ()  [unwired: 6 in, 1 out]
    }
    frame #5 {
      n461 = call "close Device.vi"("OCTDevice"=w673) -> ()  [unwired: 6 in, 1 out]
    }
    frame #6 {
      n462 = local read "AutoSafe"() -> (w674:bool)
      n463 = case shown="True" w674 {
        frame False {
        }
        frame True {
          n464 = local read "Index of Refraction"() -> (w698:dbl)
          n465 = call "get Config Path.vi"() -> ("Path"=w676:path)  [unwired: 1 in, 1 out]
          n466 = local read "Range X [mm]"() -> (w696:dbl)
          n467 = local read "Saturation"() -> (w687:sgl)
          n468 = local read "Brightness"() -> (w684:sgl)
          n469 = local read "Columns"() -> (w700:i32)
          n470 = local read "Contrast"() -> (w683:sgl)
          n471 = local read "Window"() -> (w691:T2)
          n472 = local read "Palette"() -> (w675:T1)
          n473 = Build Path(base path=w676, name or relative path=path "Settings.ini" ("Relative \"SpectralRadar.ini\" Path")) -> (appended path=w702:path)
          n474 = call "init Settings.vi"("Path to settings file"=w702) -> ("Settings"=w695:refnum<class "Settings.lvclass">)  [unwired: 5 in, 1 out]
          n475 = call "set Settings Entry Int.vi"("Value"=w700, "Node"="Columns" ("Node Name"), "Settings"=w695) -> ("Settings"=w694:refnum<class "Settings.lvclass">)  [unwired: 3 in, 1 out]
          n476 = call "set Settings Entry Float.vi"("Value"=w698, "Node"="IndexOfRefraction" ("Node Name"), "Settings"=w694) -> ("Settings"=w693:refnum<class "Settings.lvclass">)  [unwired: 3 in, 1 out]
          n477 = call "set Settings Entry Float.vi"("Value"=w696, "Node"="Range" ("Node Name"), "Settings"=w693) -> ("Settings"=w679:refnum<class "Settings.lvclass">)  [unwired: 3 in, 1 out]
          n478 = call "set Settings Entry Float.vi"("Value"=w687, "Node"="Saturation" ("Node Name"), "Settings"=w679) -> ("Settings"=w686:refnum<class "Settings.lvclass">)  [unwired: 3 in, 1 out]
          n479 = call "set Settings Entry Float.vi"("Value"=w684, "Node"="Brightness" ("Node Name"), "Settings"=w686) -> ("Settings"=w682:refnum<class "Settings.lvclass">)  [unwired: 3 in, 1 out]
          n480 = call "set Settings Entry Float.vi"("Value"=w683, "Node"="Contrast" ("Node Name"), "Settings"=w682) -> ("Settings"=w681:refnum<class "Settings.lvclass">)  [unwired: 3 in, 1 out]
          n481 = call "set Settings Entry Int.vi"("Value"=w691, "Node"="ApodizationWindow" ("Node Name"), "Settings"=w681) -> ("Settings"=w689:refnum<class "Settings.lvclass">)  [unwired: 3 in, 1 out]
          n482 = call "set Settings Entry Int.vi"("Value"=w675, "Node"="Palette" ("Node Name"), "Settings"=w689) -> ("Settings"=w678:refnum<class "Settings.lvclass">)  [unwired: 3 in, 1 out]
          n483 = call "save Settings.vi"("Settings"=w678) -> ("Settings"=w677:refnum<class "Settings.lvclass">)  [unwired: 5 in, 1 out]
          n484 = call "close Settings.vi"("Settings"=w677) -> ()  [unwired: 6 in, 1 out]
        }
      }
    }
  }
